vi "subStage_MoveRelative.vi"(7 "Stage-Ctrl":T2={"Console"={"L"=FALSE, "R"=FALSE, "FWD"=FALSE, "BACK"=FALSE}, "Step Width [mm]"=1.0, "Destination [mm]"=[6.0, 7.0], "Move "=FALSE} {"Destination [mm]" format="%_6g"; "Step Width [mm]" min=0.0 format="%_6f"}, 8 "error in":errorcluster, 10 "Stage Info":T3={" Current Position"=[-1.0, -12.0, 0.0], "Number of Axis"=3, "ILSID"=1}) -> (0 "error out":errorcluster, 5 "Console Out":T1)   [LabVIEW 2015]
panel:
  # "X"
  # "Y"
  # "X"
  # "Y"
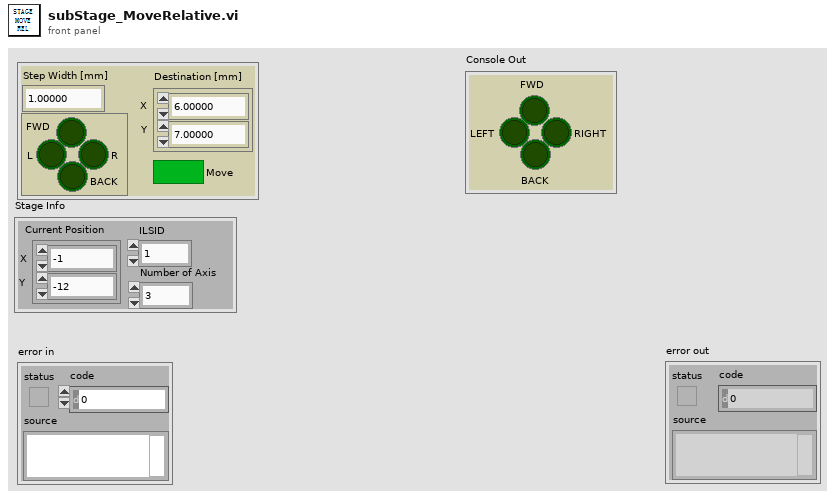
[diagram p1: front panel]
types:
  T1 = cluster{"LEFT":bool, "RIGHT":bool, "FWD":bool, "BACK":bool}
  T2 = cluster{"Console":cluster{"L":bool, "R":bool, "FWD":bool, "BACK":bool}, "Step Width [mm]":dbl, "Destination [mm]":dbl[], "Move ":bool}
  T3 = cluster{" Current Position":dbl[], "Number of Axis":i32, "ILSID":i32}
  T4 = cluster{"L":bool, "R":bool, "FWD":bool, "BACK":bool}
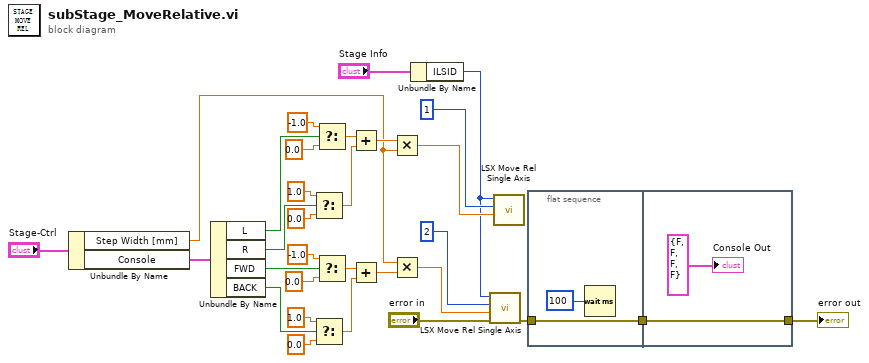
[diagram p0: block diagram]
diagram:
  n1 = Unbundle By Name("Stage-Ctrl") -> ("Step Width [mm]"=w4:dbl, "Console"=w6:T4)
  n2 = Unbundle By Name(w6) -> ("L"=w28:bool, "R"=w25:bool, "FWD"=w12:bool, "BACK"=w11:bool)
  n3 = Select(t=1.0, s=w25, f=0.0) -> (s? t:f=w23:dbl)
  n4 = Select(t=1.0, s=w11, f=0.0) -> (s? t:f=w20:dbl)
  n5 = Select(t=-1.0, s=w28, f=0.0) -> (s? t:f=w24:dbl)
  n6 = Select(t=-1.0, s=w12, f=0.0) -> (s? t:f=w19:dbl)
  n7 = Add(x=w24, y=w23) -> (x+y=w10:dbl)
  n8 = Add(x=w19, y=w20) -> (x+y=w18:dbl)
  n9 = Multiply(x=w10, y=w4) -> (x*y=w22:dbl)
  n10 = Multiply(x=w4, y=w18) -> (x*y=w21:dbl)
  n11 = Unbundle By Name("Stage Info") -> ("ILSID"=w2:i32)
  n12 = call <userlib>:"LSX Move Rel Single Axis.vi"("error in (no error)"="error in", "dValue"=w21, "lAxis"=2, "lLSID"=w2) -> ("error out"=w8:errorcluster)  [unwired: 6 in, 1 out]
  n13 = call <userlib>:"LSX Move Rel Single Axis.vi"("dValue"=w22, "lAxis"=1, "lLSID"=w2) -> ()  [unwired: 7 in, 2 out]
  n14 = flat-sequence {
    tunnel: w8 -> [w33]
    tunnel: [w33] -> w1
    tunnel: [w35] -> w7
    tunnel: w1 -> [w35]
    frame #0 {
      n15 = Wait (ms)(milliseconds to wait=u32 100) -> ()  [unwired: 1 out]
    }
    frame #1 {
      "Console Out" <- T1 {"LEFT"=FALSE, "RIGHT"=FALSE, "FWD"=FALSE, "BACK"=FALSE} ("Console")
    }
  }
  "error out" <- w7
